vi "DebugControl_Item_OnCommand.vi"(10 "Command ID":string, 11 "Object":T1) -> ()   [LabVIEW 2018]
uses:
  <resource>/Framework/Providers/API/ItemRef.ctl
panel:
  out "error out":errorcluster
  in  "error in":errorcluster
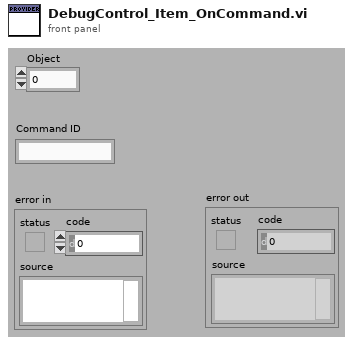
[diagram p1: front panel]
types:
  T1 = typedef "ItemRef.ctl" = u64
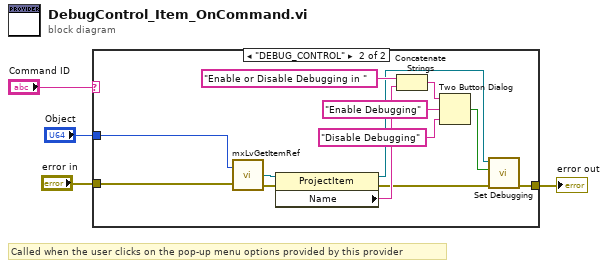
[diagram p0: block diagram]
diagram:
  # "Called when the user clicks on the pop-up menu options provided by this provider"
  n1 = case shown="\"DEBUG_CONTROL\"" "Command ID" {
    tunnel: "error in" -> [w5 w14]
    tunnel: [w5 w7] -> w2
    tunnel: "Object" -> [_ w13]
    frame Default {
    }
    frame "DEBUG_CONTROL" {
      n2 = call <resource>:"mxLvGetItemRef.vi"("Item"=w13, "error in"=w14) -> ("Item Refnum"=w18:refnum<vi>, "error out"=w17:errorcluster)  [unwired: 1 out]
      n3 = property class="ProjectItem"(reference=w18, error in=w17) -> (reference out=w9:refnum<vi>, error out=w6:errorcluster, "Name"=w15:string)
      n4 = Concatenate Strings("Enable or Disable Debugging in " ("string"), w15) -> (w12:string)
      n5 = Two Button Dialog(message=w12, 1:"Disable Debugging" ("F button name (\"Cancel\")"), 2:"Enable Debugging" ("T button name (\"OK\")")) -> (T button?=w8:bool)
      n6 = call "Set Debugging.vi"("error in (no error)"=w6, "Debugging Control"=w8, "ProjectItem in"=w9) -> ("error out"=w7:errorcluster)  [unwired: 8 in]
    }
  }
  "error out" <- w2
